vi "Pockels Cal-Detect steady state.vi"(9 "Stabil time elapsed":bool, 10 "Average V":dbl, 11 "Coeffecient of variation":dbl) -> (2 "Steady state?":bool, 3 "Weighted COV":dbl format="%#.4f")   [LabVIEW 2020]
panel:
  in  "COV +/- pass range":dbl=0.3 format="%#_13g"
  in  "Weighted COV +/- pass range":dbl=0.03 format="%#_13g"
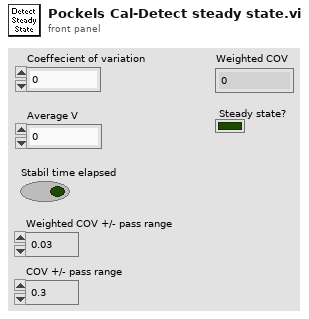
[diagram p1: front panel]
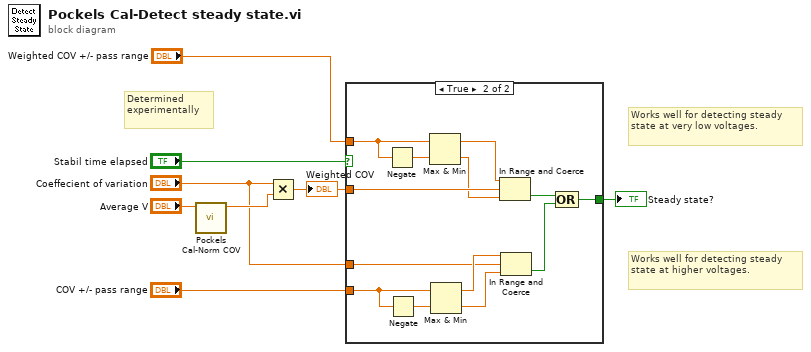
[diagram p0: block diagram]
diagram:
  # "Works well for detecting steady state at higher voltages."
  # "Works well for detecting steady state at very low voltages."
  # "Determined experimentally"
  n1 = call "Pockels Cal-Norm COV.vi"("Coeffecient of variation"="Average V") -> ("Weighting (rormalised V)"=w7:dbl)  [unwired: 10 in]
  n2 = Multiply(x="Coeffecient of variation", y=w7) -> (x*y=w8:dbl)
  "Weighted COV" <- w8
  n3 = case shown="True" "Stabil time elapsed" {
    tunnel: w8 -> [_ w21]
    tunnel: [_ w10] -> w5
    tunnel: "Weighted COV +/- pass range" -> [_ w19]
    tunnel: "COV +/- pass range" -> [_ w13]
    tunnel: "Coeffecient of variation" -> [_ w12]
    frame False {
    }
    frame True {
      n4 = Negate(x=w19) -> (-x=w20:dbl)
      n5 = Negate(x=w13) -> (-x=w14:dbl)
      n6 = Max & Min(x=w19, y=w20) -> (max(x,y)=w18:dbl, min(x,y)=w17:dbl)
      n7 = Max & Min(x=w13, y=w14) -> (max(x,y)=w15:dbl, min(x,y)=w16:dbl)
      n8 = In Range and Coerce(upper limit=w18, x=w21, lower limit=w17) -> (In Range?=w11:bool)  [unwired: 1 out]
      n9 = In Range and Coerce(upper limit=w15, x=w12, lower limit=w16) -> (In Range?=w9:bool)  [unwired: 1 out]
      n10 = Compound Arithmetic op=OR(w11, w9) -> (w10:bool)
    }
  }
  "Steady state?" <- w5
